vi "sub_master_joystick-info_strconv.vi"(11 "velocity":cluster{dbl, dbl} {"?" format="%.7f"; "?" format="%.7f"}) -> (3 "str out":string)   [LabVIEW 2019]
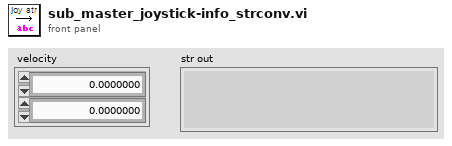
[diagram p1: front panel]
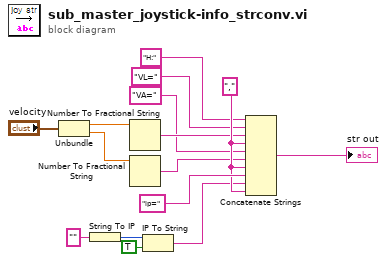
[diagram p0: block diagram]
diagram:
  w14 = ","
  n1 = Unbundle("velocity") -> (w5:dbl, w4:dbl)
  n2 = String To IP(1:"" ("name")) -> (0:w11:u32)
  n3 = Number To Fractional String(number=w5) -> (F-format string=w7:string)  [unwired: 3 in]
  n4 = Number To Fractional String(number=w4) -> (F-format string=w6:string)  [unwired: 3 in]
  n5 = IP To String(1:TRUE ("dot notation? (F)"), 2:w11) -> (0:w13:string)
  n6 = Concatenate Strings("H:", "VL=", w7, w14, "VA=", w6, w14, "ip=", w13, w14) -> (→"str out":string)
